vi "FeedbackDecode_CustomRaster.vi"(0 "StitchArray":dbl[][](array[numeric]), 1 "Fs":dbl=1000.0, 2 "RstrCtrl":T1={"RstrScl"=1.0, "RstrZoom"=0.0, "RstrOffset"=0.0, "RstrTime"=10000} {"RstrTime" min=100 max=10000 step=1; "RstrOffset" min=1.0 step=1.0; "RstrZoom" min=0.0 step=0.1; "RstrScl" min=1.0 step=0.1}, 3 "FiltSpec":T2={"Topology"=enum."Off", "Type"=enum."Lowpass", "#Taps"=50, "Lower PB"=100.0, "Upper PB"=0.0, "Lower SB"=200.0, "Upper SB"=0.0} {"Lower SB" format="%0.2p"; "Upper SB" format="%0.2p"; "Lower PB" format="%0.2p"; "Upper PB" format="%0.2p"}, 5 "RBuffSize":i32=1000 caption="Window Size" min=100 max=10000 step=1) -> (6 "CurIdx":i32=1, 8 "RasterOut":dbl[][](array[numeric]))   [LabVIEW 2020]
uses:
  <vilib>/measure/macond.llb/FIR Filter for N Chan.vi
  <vilib>/measure/NI_MAPro.lvlib
panel:
  in  "TotIdx":i32=1
  in  "RasterBuff":dbl[][](array[numeric])
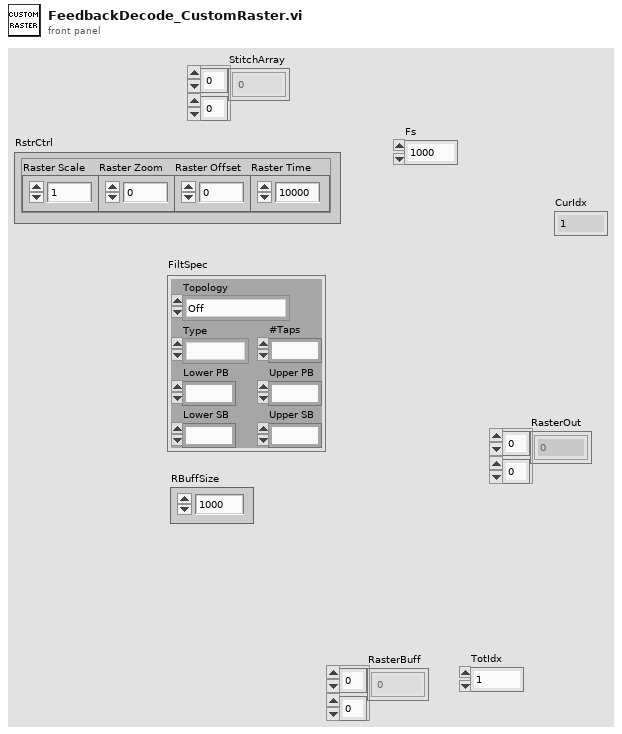
[diagram p1: front panel]
types:
  T1 = cluster{"RstrScl":dbl, "RstrZoom":dbl, "RstrOffset":dbl, "RstrTime":i32}
  T2 = cluster{"Topology":enum16{"Off", "FIR by Specification", "Equi-ripple FIR", "Windowed FIR"}, "Type":enum16{"Lowpass", "Highpass", "Bandpass", "Bandstop"}, "#Taps":i32, "Lower PB":dbl, "Upper PB":dbl, "Lower SB":dbl, "Upper SB":dbl}
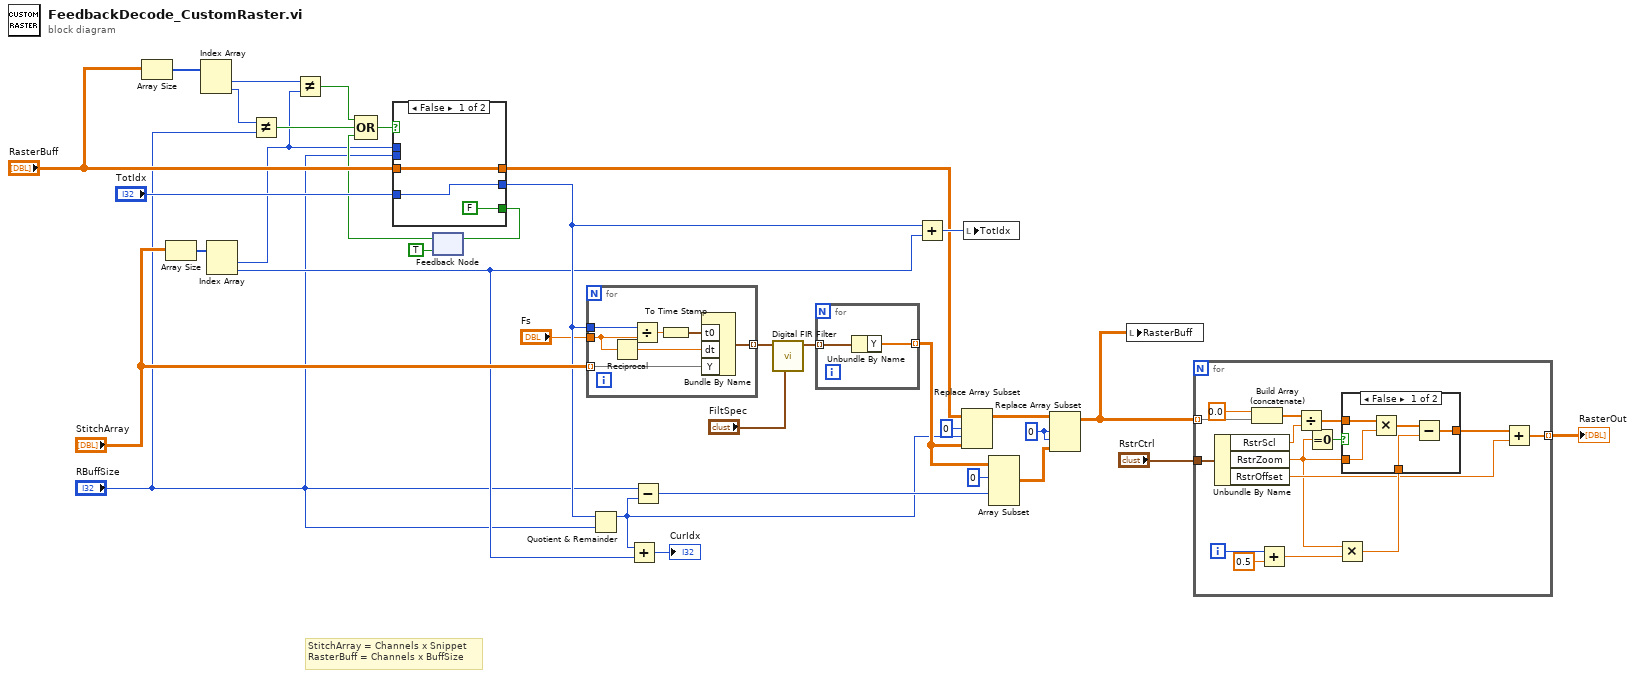
[diagram p0: block diagram]
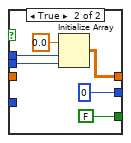
[diagram p3: hidden frame]
diagram:
  w28 = 0 ("disabled index (col)")
  # "StitchArray = Channels x Snippet\nRasterBuff = Channels x BuffSize"
  n1 = Array Size(array="RasterBuff") -> (size(s)=w8:i32[])
  n2 = Array Size(array="StitchArray") -> (size(s)=w9:i32[])
  n3 = Index Array(array=w8) -> (element #1=w4:i32, element #2=w6:i32)  [unwired: 2 in]
  n4 = Index Array(array=w9) -> (element #1=w3:i32, element #2=w10:i32)  [unwired: 2 in]
  n5 = Not Equal?(x=w6, y="RBuffSize") -> (x != y?=w5:bool)
  n6 = Not Equal?(x=w4, y=w3) -> (x != y?=w2:bool)
  n7 = feedback #1(TRUE) -> (w16:bool)
  n8 = Compound Arithmetic op=OR(w2, w5, w16) -> (w17:bool)
  n9 = case shown="False" w17 {
    tunnel: [w38 w43] -> w33
    tunnel: "RBuffSize" -> [_ w41]
    tunnel: "RasterBuff" -> [w38 _]
    tunnel: "TotIdx" -> [w37 _]
    tunnel: [w37 0 ("CurIdx")] -> w18
    tunnel: w3 -> [_ w40]
    tunnel: [FALSE FALSE] -> w14
    frame False {
    }
    frame True {
      n10 = Initialize Array(0.0 ("element"), w40, w41) -> (w43:dbl[][])
    }
  }
  n11 = feedback-in #1(w14) -> ()
  n12 = for {
    tunnel: w18 -> [w51]
    tunnel: "StitchArray" -> [w48] mode=indexing
    tunnel: [w47] -> w23 mode=indexing
    tunnel: "Fs" -> [w46]
    n13 = Reciprocal(x=w46) -> (1/x=w45:dbl)
    n14 = Divide(x=w51, y=w46) -> (x/y=w50:dbl)
    n15 = To Time Stamp(1:w50) -> (0:w49:timestamp)
    n16 = Bundle By Name("t0"=w49, "dt"=w45, "Y"=w48) -> (w47:waveform(dbl))  [unwired: 1 in]
  }
  n17 = Quotient & Remainder(x=w18, y="RBuffSize") -> (x-y*floor(x/y)=w12:i32)  [unwired: 1 out]
  n18 = Add(x=w12, y=w10) -> (x+y=→"CurIdx":i32)
  n19 = Subtract(x="RBuffSize", y=w12) -> (x-y=w31:i32)
  n20 = call-poly <vilib>:"Digital FIR Filter.vi"("FIR filter specifications"="FiltSpec", "signal(s) in"=w23) -> ("signal(s) out"=w22:waveform(dbl)[])  [unwired: 7 in, 2 out]
  n21 = for {
    tunnel: w22 -> [w53] mode=indexing
    tunnel: [w52] -> w21 mode=indexing
    n22 = Unbundle By Name(w53) -> ("Y"=w52:dbl[])
  }
  n23 = Add(x=w18, y=w10) -> (x+y=w35:i32)
  n24 = Replace Array Subset(array=w33, new element=w21, index (row)=0 ("disabled index (row)"), index (col)=w12) -> (w26:dbl[][])
  n25 = local write "TotIdx"(w35) -> ()
  n26 = Array Subset(array=w21, index (row)=0 ("index"), index (col)=w31) -> (w27:dbl[][])  [unwired: 2 in]
  n27 = Replace Array Subset(array=w26, new element=w27, index (row)=w28, index (col)=w28) -> (w19:dbl[][])
  n28 = local write "RasterBuff"(w19) -> ()
  n29 = for {
    tunnel: w19 -> [w58] mode=indexing
    tunnel: [w60] -> w20 mode=indexing
    tunnel: "RstrCtrl" -> [w67]
    i -> [w64]
    n30 = Unbundle By Name(w67) -> ("RstrScl"=w66:dbl, "RstrZoom"=w54:dbl, "RstrOffset"=w59:dbl)
    n31 = Build Array (concatenate)(0.0, w58) -> (w57:dbl[])
    n32 = Add(x=w64, y=0.5) -> (x+y=w62:dbl)
    n33 = Divide(x=w57, y=w66) -> (x/y=w65:dbl[])
    n34 = Equal To 0?(x=w54) -> (x = 0?=w55:bool)
    n35 = Multiply(x=w54, y=w62) -> (x*y=w68:dbl)
    n36 = case shown="False" w55 {
      tunnel: w68 -> [w73 _]
      tunnel: w65 -> [w72 w74]
      tunnel: [w70 w74] -> w61
      tunnel: w54 -> [w69 _]
      frame False {
        n37 = Multiply(x=w72, y=w69) -> (x*y=w71:dbl[])
        n38 = Subtract(x=w71, y=w73) -> (x-y=w70:dbl[])
      }
      frame True {
      }
    }
    n39 = Add(x=w61, y=w59) -> (x+y=w60:dbl[])
  }
  "RasterOut" <- w20
